vi "Parse Signed Identifier.vi"(11 "String":string) -> (3 "Signed identifier":T1)   [LabVIEW 2015, in "NI_Azure_Queue.lvlib"]
uses:
  NI_Azure_Queue.lvlib
  Signed Identifier.ctl
  Access Policy.ctl
  XML Parsing/NI_Azure_XML Parsing.lvlib
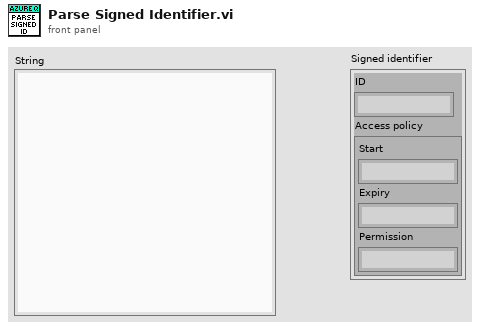
[diagram p1: front panel]
types:
  T1 = typedef "NI_Azure_Queue.lvlib/Signed Identifier.ctl" = cluster{"ID":string, "Access policy":T2}
  T2 = typedef "NI_Azure_Queue.lvlib/Access Policy.ctl" = cluster{"Start":string, "Expiry":string, "Permission":string}
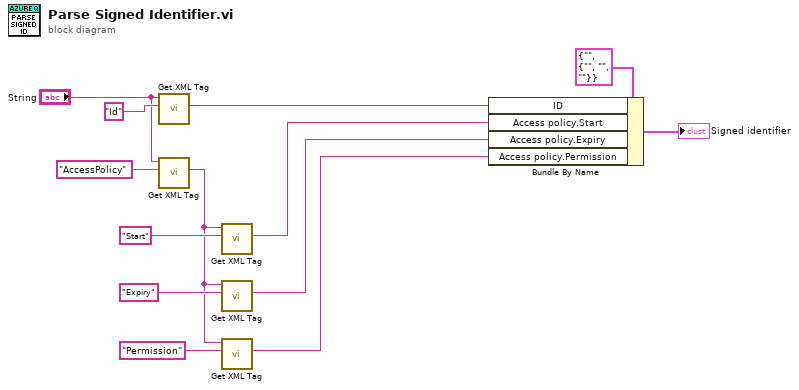
[diagram p0: block diagram]
diagram:
  n1 = call "Get XML Tag.vi"("Tag name"="Id", "XML String in"="String") -> ("Tag value"=w4:string)  [unwired: 5 in, 4 out]
  n2 = call "Get XML Tag.vi"("Tag name"="AccessPolicy", "XML String in"="String") -> ("Tag value"=w7:string)  [unwired: 5 in, 4 out]
  n3 = call "Get XML Tag.vi"("Tag name"="Start", "XML String in"=w7) -> ("Tag value"=w3:string)  [unwired: 5 in, 4 out]
  n4 = call "Get XML Tag.vi"("Tag name"="Expiry", "XML String in"=w7) -> ("Tag value"=w2:string)  [unwired: 5 in, 4 out]
  n5 = call "Get XML Tag.vi"("Tag name"="Permission", "XML String in"=w7) -> ("Tag value"=w1:string)  [unwired: 5 in, 4 out]
  n6 = Bundle By Name(cluster=T1 {"ID"="", "Access policy"={"Start"="", "Expiry"="", "Permission"=""}} ("Signed identifier"), "ID"=w4, "Access policy.Start"=w3, "Access policy.Expiry"=w2, "Access policy.Permission"=w1) -> (→"Signed identifier":T1)
